vi "IMAQ HL-Snap.vi"(7 "ImgName":string="untitled", 8 "ErrIn":errorcluster, 11 "IF Name":string="img0") -> (0 "ErrOut":errorcluster, 3 "ImgOut":T1)   [LabVIEW 2016]
doc: "Use this template to build a VI to use as a subVI."
uses:
  <vilib>/vision/Image Controls.llb/IMAQ Image.ctl
panel:
  # "Input Parameters"
  # "Output Parameters"
  # "VI Description:\nThis VI is created to snap a image from imaging device."
  # ":: MVI Framework V1.0 ::\nAuthor:Gaoke Yang\nEmail: gaoke.yang@yahoo.com\nWeb: www.mvicontrol.com\nCopyright (C) 2013, MVI Technologies All Rights Reserved"
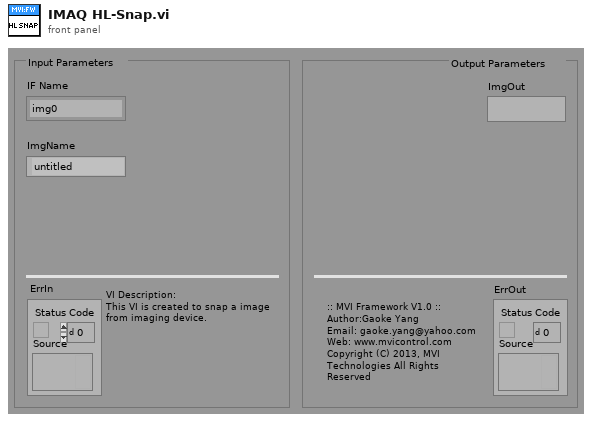
[diagram p1: front panel]
types:
  T1 = typedef "IMAQ Image.ctl" = refnum<image>
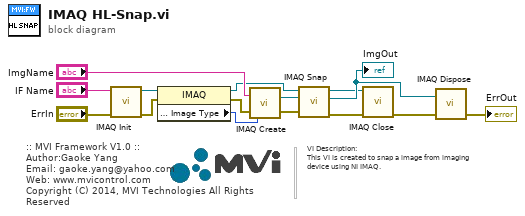
[diagram p0: block diagram]
diagram:
  # "VI Description:\nThis VI is created to snap a image from imaging\ndevice using NI IMAQ."
  # ":: MVI Framework V1.0 ::\nAuthor:Gaoke Yang\nEmail: gaoke.yang@yahoo.com\nWeb: www.mvicontrol.com\nCopyright (C) 2014, MVI Technologies All Rights Reserved"
  n1 = call <vilib>:"IMAQ Init.vi"("error in (no error)"="ErrIn", "Interface Name"="IF Name") -> ("error out"=w8:errorcluster, "IMAQ Session Out"=w9:refnum<k11>)  [unwired: 8 out]
  n2 = property class="IMAQ"(reference=w9, error in=w8) -> (reference out=w6:refnum<k11>, error out=w7:errorcluster, "Image Parameters : Image Type"=w5:u32)
  n3 = call "IMAQ Create"("Image Name"="ImgName", "Image Type"=w5, "error in (no error)"=w7) -> ("New Image"=w10:T1, "error out"=w4:errorcluster)  [unwired: 1 in, 1 out]
  n4 = call <vilib>:"IMAQ Snap.vi"("error in (no error)"=w4, "Image In"=w10, "IMAQ Session In"=w6) -> ("error out"=w1:errorcluster, "Image Out"=w11:T1, "IMAQ Session Out"=w2:refnum<k11>)  [unwired: 6 out]
  "ImgOut" <- w11
  n5 = call <vilib>:"IMAQ Close.vi"("error in (no error)"=w1, "IMAQ Session In"=w2) -> ("error out"=w3:errorcluster)  [unwired: 9 out]
  n6 = call "IMAQ Dispose"("Image"=w11, "error in (no error)"=w3) -> ("error out"=→"ErrOut":errorcluster)  [unwired: 1 in, 3 out]
